vi "TestAdministrator.vi"() -> ()   [LabVIEW 2017]
doc: "Test executive administrator."
uses:
  Shared/Support_InvocationInfo.ctl
panel:
  out "error out":errorcluster
  out "Allocated Memory":T1(graph)
  out "PASS":bool
  in  "Unload after sequence done?":bool
  out "Sequence start time":string
  in  "Only save fails?":bool
  out "# of steps PASSED":i32
  out "# of steps executed":i32
  out "Result file":path
  out "Loop index":i32
  out "Running":bool
  in  "exit":bool
  in  "stop":bool
  out "Last step result":string
  in  "Run":bool
  in  "Nr of loops":i32=1
  in  "Loop infinitive?":bool
  in  "Save to result file?":bool=TRUE
  in  "Result folder":path=path "C:/Users/materi/Documents/G#"
  in  "Load":bool
  in  "Test case folder":path=path "C:/Projects/GsharpGIT2017/Verification/TestCases"
  in  "Sequence file":path=path "C:/Projects/GsharpGIT2017/Verification/TestCases/KernelTestSequence.seq"
  out "Steps":i32(listbox)
  # "Test Administrator"
  # "Execution"
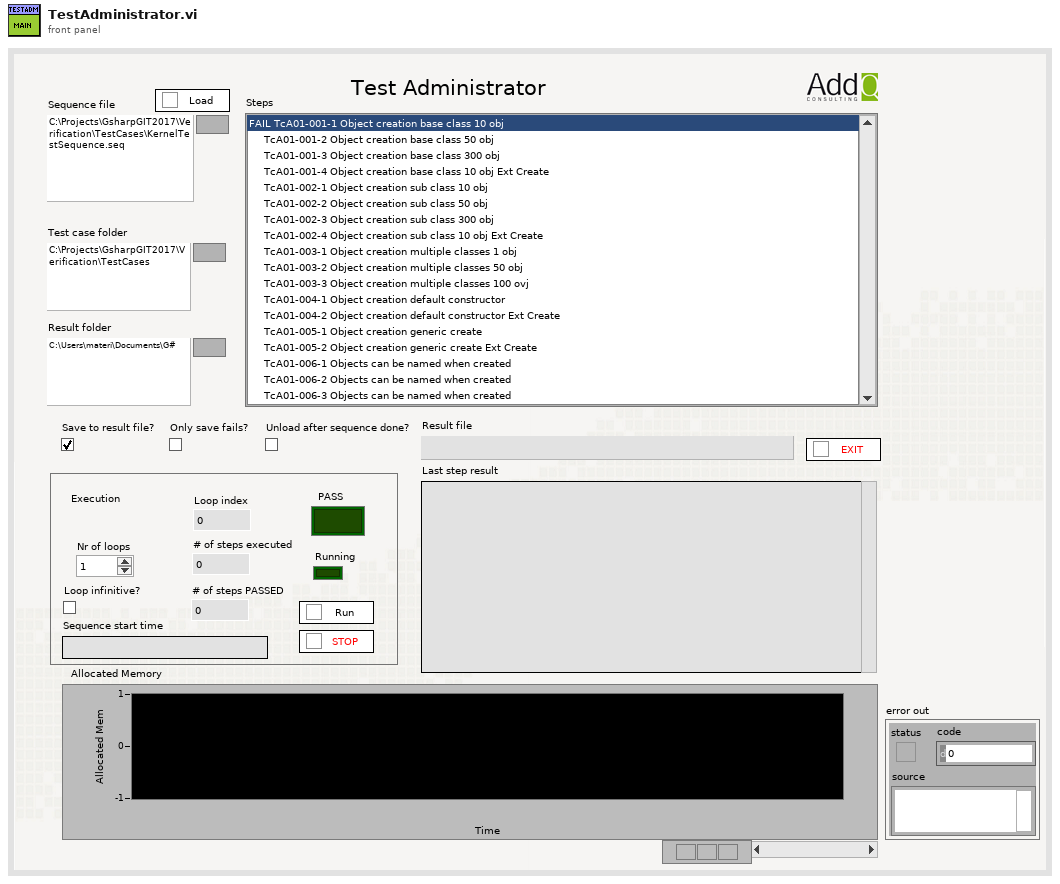
[diagram p1: front panel]
types:
  T1 = cluster{"seconds since 1Jan1904":timestamp, "totAllocSize":i64}[]
  T2 = cluster{"Step names":string[], "Step VIs":string[], "Input Buffer":string[], "Step VI paths":path[], "Loop infinite":bool, "Sequence start time":string, "Save to result file?":bool, "Result file":refnum<file>, "File index":i32, "Nr of PASS":i32, "Nr of steps":i32}
  T3 = enum16{"open", "open or create", "create or replace", "create", "open (read only)"}
  T4 = typedef "Support_InvocationInfo.ctl" = cluster{"UUT #":i32, "loop #":i32, "UUT Info":string, "Test Name":string, "Sequence Path":path}
  T5 = cluster{"PASS/FAIL Flag":bool, "Numeric Measurement":dbl, "String Measurement":string, "Report Text":string}
  T6 = cluster{"totalFreeSize":i64, "maxFreeSize":i64, "nFreeblocks":i64, "totAllocSize":i64, "maxAllocSize":i64, "nPointers":i64, "nUnlockedHdls":i64, "nLockedHdls":i64, "reserved1":i32, "reserved2":i32, "reserved3":i32, "reserved4":i32}
  T7 = cluster{"seconds since 1Jan1904":timestamp, "totAllocSize":i64}
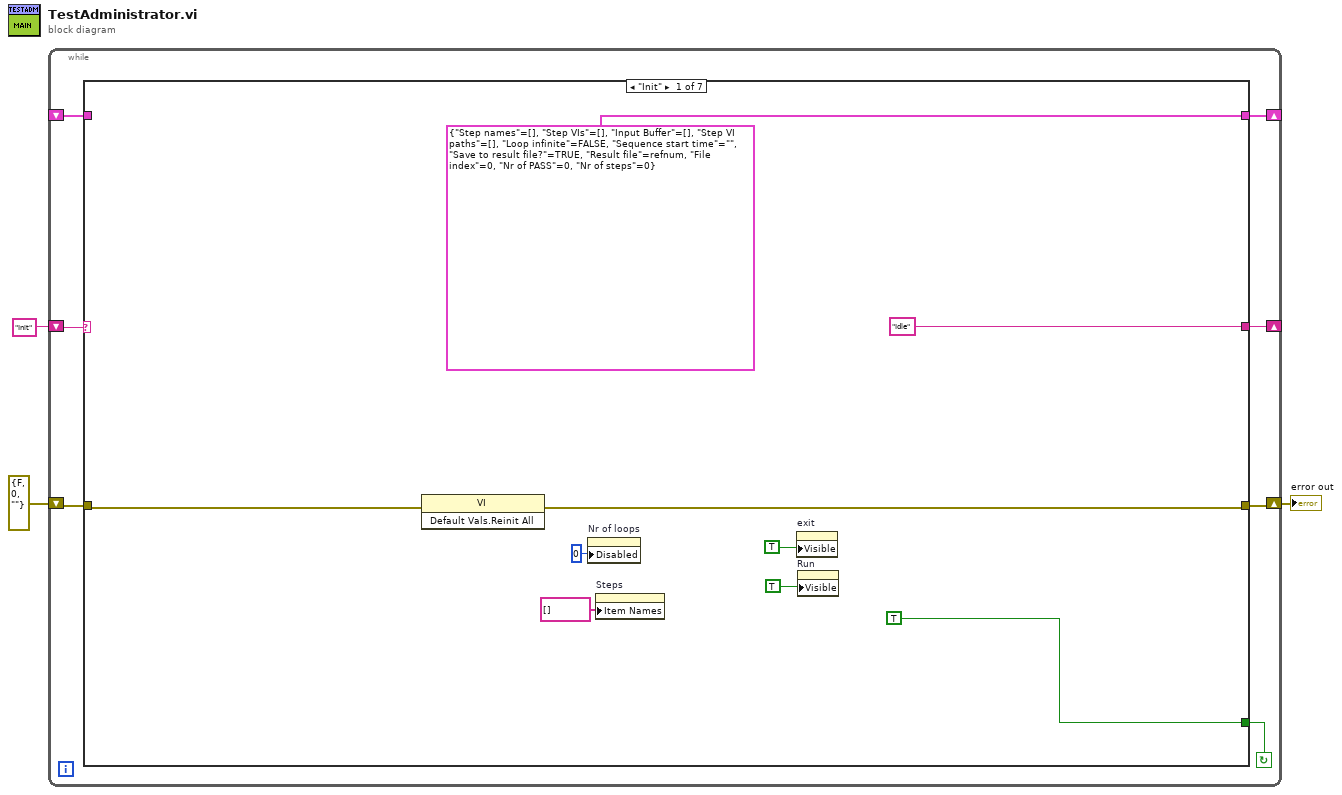
[diagram p0: block diagram]
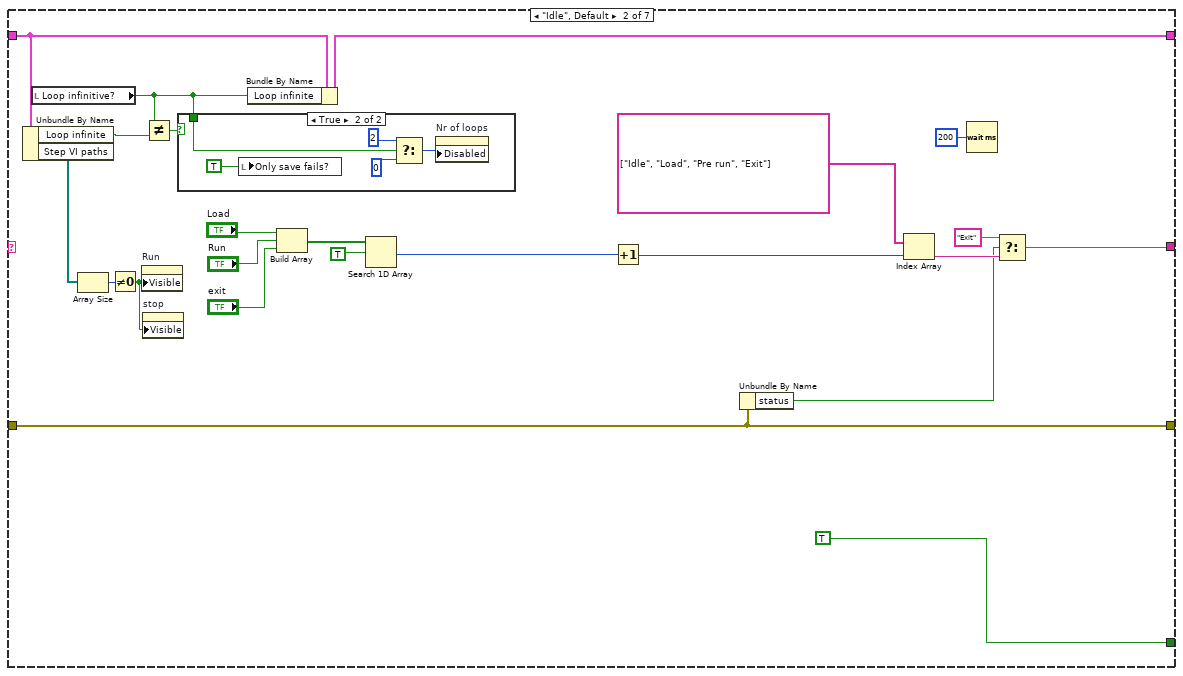
[diagram p2: hidden frame]
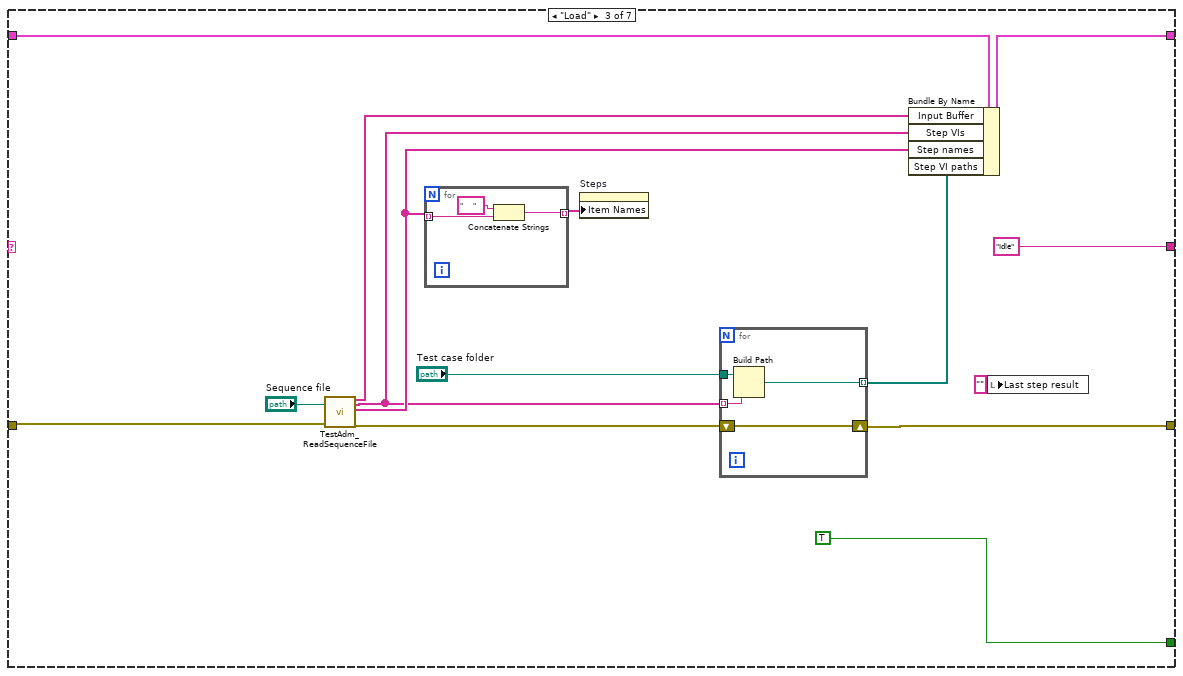
[diagram p4: hidden frame]
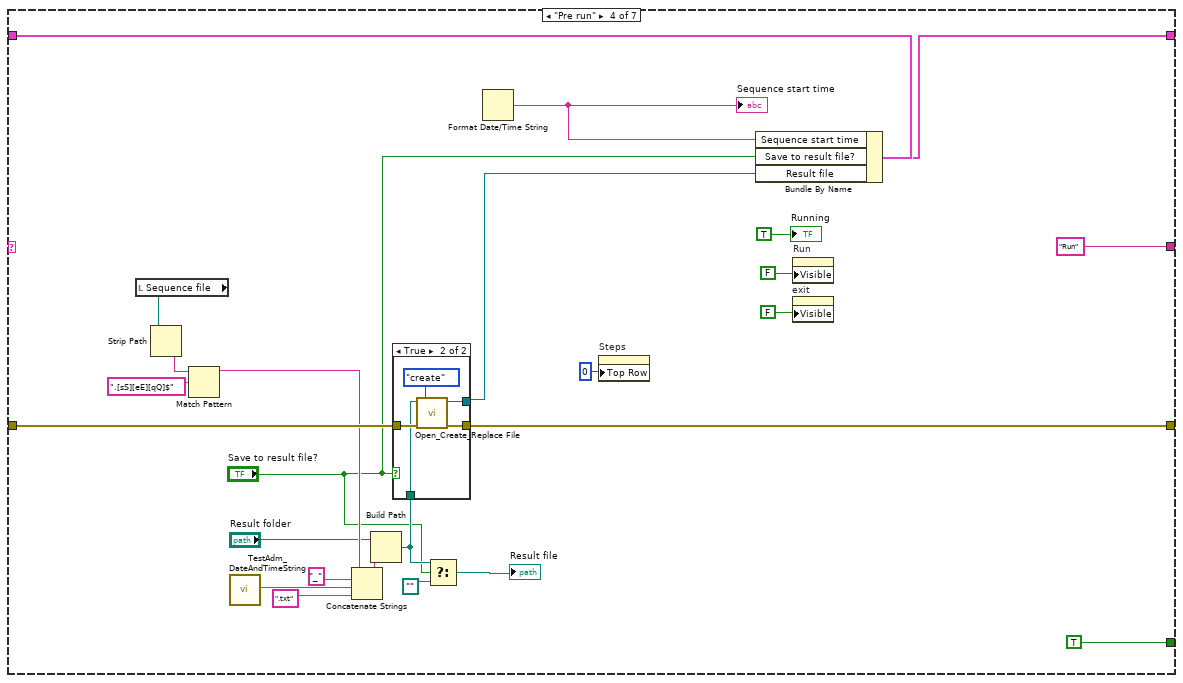
[diagram p5: hidden frame]
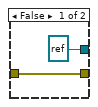
[diagram p6: hidden frame]
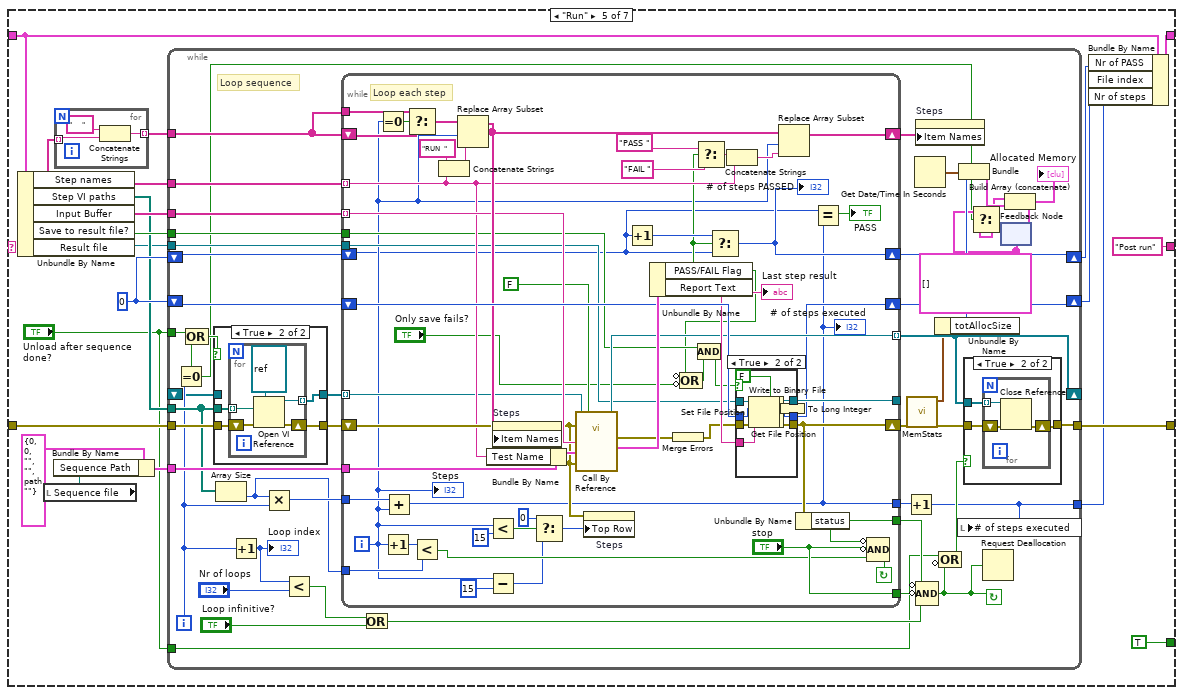
[diagram p7: hidden frame]
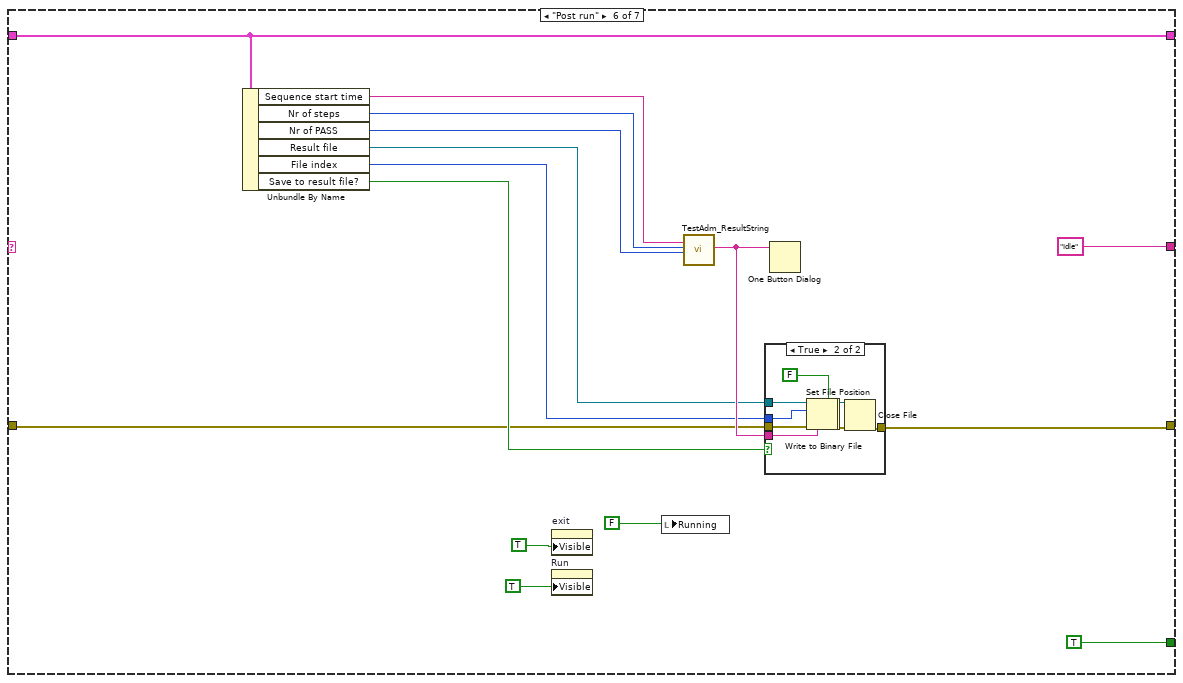
[diagram p11: hidden frame]
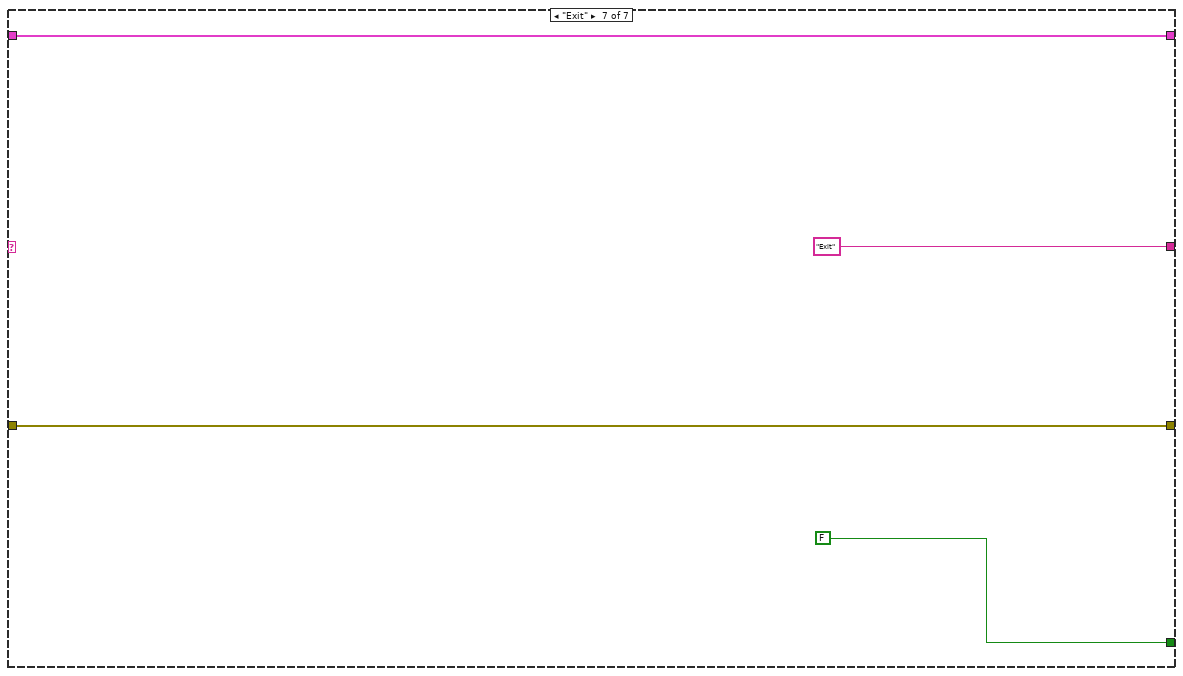
[diagram p13: hidden frame]
diagram:
  n1 = while {
    shift-left: errorcluster {"status"=FALSE, "code"=0, "source"=""} ("error out") -> [w8]
    shift-right: [w7] -> w1
    shift-left: _ -> [w6]
    shift-right: [w9] -> _
    shift-left: "Init" -> [w10]
    shift-right: [w5] -> _
    stop <- w4 continue-if-true
    n2 = case shown="\"Init\"" w10 {
      tunnel: [T2 {"Step names"=[], "Step VIs"=[], "Input Buffer"=[], "Step VI paths"=[], "Loop infinite"=FALSE, "Sequence start time"="", "Save to result file?"=TRUE, "Result file"=refnum, "File index"=0, "Nr of PASS"=0, "Nr of steps"=0} w26 w61 w77 w110 w267 w286] -> w9
      tunnel: w8 -> [w17 w31 w49 w92 w113 w262 w285]
      tunnel: [w16 w31 w56 w79 w112 w269 w285] -> w7
      tunnel: w6 -> [_ w27 w57 w78 w111 w267 w286]
      tunnel: ["Idle" w34 "Idle" "Run" ("t") "Post run" ("t") "Idle" ("t") "Exit" ("t")] -> w5
      tunnel: [TRUE TRUE TRUE TRUE TRUE TRUE FALSE] -> w4
      frame "Init" {
        n3 = invoke class="VI" method="Default Vals.Reinit All"(error in=w17) -> (error out=w16:errorcluster)  [unwired: 2 in, 2 out]
        n4 = property on="Nr of loops" class="DigNum (strict)"("Disabled"=u8 0) -> ()  [unwired: 2 in, 2 out]
        n5 = property on="Steps" class="LstBox (strict)"("Item Names"=string[] []) -> ()  [unwired: 2 in, 2 out]
        n6 = property on="exit" class="Bool"("Visible"=TRUE) -> ()  [unwired: 2 in, 2 out]
        n7 = property on="Run" class="Bool"("Visible"=TRUE) -> ()  [unwired: 2 in, 2 out]
      }
      frame "Idle", Default {
        n8 = Unbundle By Name(w27) -> ("Loop infinite"=w25:bool, "Step VI paths"=w23:path[])
        n9 = local read "Loop infinitive?"() -> (w20:bool)
        n10 = Array Size(array=w23) -> (size(s)=w22:i32)
        n11 = Not Equal To 0?(x=w22) -> (x != 0?=w21:bool)
        n12 = property on="Run" class="Bool"("Visible"=w21) -> ()  [unwired: 2 in, 2 out]
        n13 = property on="stop" class="Bool"("Visible"=w21) -> ()  [unwired: 2 in, 2 out]
        n14 = Not Equal?(x=w20, y=w25) -> (x != y?=w24:bool)
        n15 = case shown="True" w24 {
          tunnel: w20 -> [_ w46]
          frame False {
          }
          frame True {
            n16 = local write "Only save fails?"(TRUE ("Save to result file?")) -> ()
            n17 = Select(t=u8 2 ("Disabled"), s=w46, f=u8 0 ("Disabled")) -> (s? t:f=w43:u8)
            n18 = property on="Nr of loops" class="DigNum (strict)"("Disabled"=w43) -> ()  [unwired: 2 in, 2 out]
          }
        }
        n19 = Bundle By Name(cluster=w27, "Loop infinite"=w20) -> (w26:T2)
        n20 = Build Array("Load", "Run", "exit") -> (w35:bool[])
        n21 = Search 1D Array(1D array=w35, element=TRUE) -> (index of element=w40:i32)  [unwired: 1 in]
        n22 = Increment(x=w40) -> (x+1=w41:i32)
        n23 = Unbundle By Name(w31) -> ("status"=w30:bool)
        n24 = Index Array(array=string[] ["Idle", "Load", "Pre run", "Exit"] ("Array Constant"), index=w41) -> (element=w33:string)
        n25 = Wait (ms)(milliseconds to wait=u32 200) -> ()  [unwired: 1 out]
        n26 = Select(t="Exit", s=w30, f=w33) -> (s? t:f=w34:string)
      }
      frame "Load" {
        n27 = call "TestAdm_ReadSequenceFile.vi"("Path"="Sequence file", "error in (no error)"=w49) -> ("Input Buffer"=w60:string[], "Step paths"=w50:string[], "Step names"=w52:string[], "error out"=w55:errorcluster)  [unwired: 14 in]
        n28 = for {
          tunnel: [w63] -> w53 mode=indexing
          tunnel: w52 -> [w65] mode=indexing
          n29 = Concatenate Strings("     " ("Substring"), w65) -> (w63:string)
        }
        n30 = property on="Steps" class="LstBox (strict)"("Item Names"=w53) -> ()  [unwired: 2 in, 2 out]
        n31 = for {
          shift-right: [w67] -> w56
          shift-left: w55 -> [w67]
          tunnel: "Test case folder" -> [w69]
          tunnel: w50 -> [w68] mode=indexing
          tunnel: [w66] -> w48 mode=indexing
          n32 = Build Path(base path=w69, name or relative path=w68) -> (appended path=w66:path)
        }
        n33 = Bundle By Name(cluster=w57, "Input Buffer"=w60, "Step VIs"=w50, "Step names"=w52, "Step VI paths"=w48) -> (w61:T2)
        n34 = local write "Last step result"("" ("Last Step result")) -> ()
      }
      frame "Pre run" {
        n35 = local read "Sequence file"() -> (w87:path)
        n36 = Strip Path(path=w87) -> (name=w86:string)  [unwired: 1 out]
        n37 = Match Pattern(string=w86, regular expression=".[sS][eE][qQ]$") -> (before substring=w85:string)  [unwired: 1 in, 3 out]
        n38 = call "TestAdm_DateAndTimeString.vi"() -> ("String out"=w91:string)  [unwired: 19 in]
        n39 = Concatenate Strings(w85, "_", w91, ".txt" ("Substring")) -> (w90:string)
        n40 = Build Path(base path="Result folder", name or relative path=w90) -> (appended path=w89:path)
        n41 = case shown="True" "Save to result file?" {
          tunnel: w92 -> [w96 w101]
          tunnel: [refnum<file> refnum ("refnum") w100] -> w74
          tunnel: [w96 w99] -> w79
          tunnel: w89 -> [_ w97]
          frame False {
          }
          frame True {
            n42 = call <vilib>:"Open_Create_Replace File.vi"("error in (no error)"=w101, "function (open:0)"=T3."create", "file path"=w97) -> ("error out"=w99:errorcluster, "refnum"=w100:refnum<file>)  [unwired: 5 in, 2 out]
          }
        }
        n43 = Select(t=w89, s="Save to result file?", f=path "") -> (s? t:f=→"Result file":path)
        n44 = Format Date/Time String() -> (date/time string=w76:string)  [unwired: 3 in]
        "Sequence start time" <- w76
        n45 = property on="Steps" class="LstBox (strict)"("Top Row"=0) -> ()  [unwired: 2 in, 2 out]
        n46 = Bundle By Name(cluster=w78, "Sequence start time"=w76, "Save to result file?"="Save to result file?", "Result file"=w74) -> (w77:T2)
        n47 = property on="Run" class="Bool"("Visible"=FALSE) -> ()  [unwired: 2 in, 2 out]
        n48 = property on="exit" class="Bool"("Visible"=FALSE) -> ()  [unwired: 2 in, 2 out]
        "Running" <- TRUE ("Running")
      }
      frame "Run" {
        w107 = 0 ("offset")
        n49 = Unbundle By Name(w111) -> ("Step names"=w117:string[], "Step VI paths"=w106:path[], "Input Buffer"=w109:string[], "Save to result file?"=w114:bool, "Result file"=w105:refnum<file>)
        n50 = local read "Sequence file"() -> (w115:path)
        n51 = Bundle By Name(cluster=T4 {"UUT #"=0, "loop #"=0, "UUT Info"="", "Test Name"="", "Sequence Path"=path ""} ("Invocation info"), "Sequence Path"=w115) -> (w118:T4)
        n52 = for {
          tunnel: w117 -> [w258] mode=indexing
          tunnel: [w256] -> w116 mode=indexing
          n53 = Concatenate Strings("     ", w258) -> (w256:string)
        }
        n54 = while {
          tunnel: [w134] -> w102
          shift-left: _ -> [w137]
          shift-right: [w136] -> _
          tunnel: "Unload after sequence done?" -> [w138]
          tunnel: "Unload after sequence done?" -> [w139]
          tunnel: w105 -> [w154]
          tunnel: w106 -> [w153]
          shift-left: w107 -> [w158]
          shift-right: [w160] -> w108
          shift-left: w107 -> [w159]
          shift-right: [w161] -> w103
          tunnel: [w142] -> w112
          tunnel: w113 -> [w156]
          tunnel: w114 -> [w162]
          tunnel: w116 -> [w163]
          tunnel: w117 -> [w164]
          tunnel: w109 -> [w166]
          tunnel: w118 -> [w167]
          i -> [w141]
          stop <- w130 continue-if-true
          w125 = T1 []
          # "Loop sequence"
          n55 = Equal To 0?(x=w141) -> (x = 0?=w122:bool)
          n56 = Compound Arithmetic op=OR(w139, w122) -> (w140:bool)
          n57 = case shown="True" w140 {
            tunnel: [w246 w250] -> w157
            tunnel: w156 -> [w246 w249]
            tunnel: [w245 w248] -> w155
            tunnel: w153 -> [_ w247]
            tunnel: w137 -> [w245 _]
            frame False {
            }
            frame True {
              n58 = for {
                shift-right: [w254] -> w250
                shift-left: w249 -> [w255]
                tunnel: [w252] -> w248 mode=indexing
                tunnel: w247 -> [w251] mode=indexing
                n59 = Open VI Reference(type specifier VI Refnum (for type only)=refnum<vi> refnum ("VI Refnum"), vi path=w251, error in (no error)=w255) -> (vi reference=w252:refnum<vi>, error out=w254:errorcluster)  [unwired: 3 in]
              }
            }
          }
          n60 = Array Size(array=w153) -> (size(s)=w148:i32)
          n61 = Increment(x=w141) -> (x+1=w147:i32)
          "Loop index" <- w147
          n62 = Multiply(x=w148, y=w141) -> (x*y=w152:i32)
          n63 = Less?(x=w147, y="Nr of loops") -> (x < y?=w145:bool)
          n64 = while {
            tunnel: w148 -> [w189]
            tunnel: ["stop"] -> w149
            tunnel: [w221] -> w150
            tunnel: [w171] -> w151
            tunnel: w152 -> [w191]
            tunnel: w154 -> [w192]
            tunnel: [w193] -> w136 mode=indexing
            tunnel: w155 -> [w194] mode=indexing
            tunnel: w163 -> [w199]
            shift-left: w159 -> [w169]
            shift-right: [w173] -> w161
            shift-left: w163 -> [w200]
            shift-right: [w214] -> w165
            tunnel: w164 -> [w195] mode=indexing
            tunnel: [w215] -> _
            shift-left: w158 -> [w217]
            shift-right: [w172] -> w160
            tunnel: w162 -> [w178]
            tunnel: w166 -> [w196] mode=indexing
            tunnel: w167 -> [w209]
            shift-left: w157 -> [w204]
            shift-right: [w218] -> w133
            i -> [w170]
            stop <- w220 continue-if-true
            # "Loop each step"
            n65 = Equal To 0?(x=w170) -> (x = 0?=w197:bool)
            n66 = Increment(x=w170) -> (x+1=w175:i32)
            n67 = Add(x=w191, y=w170) -> (x+y=w171:i32)
            "# of steps executed" <- w171
            n68 = Select(t=w199, s=w197, f=w200) -> (s? t:f=w198:string[])
            n69 = Less?(x=w175, y=w189) -> (x < y?=w188:bool)
            n70 = Concatenate Strings("RUN  ", w195) -> (w205:string)
            n71 = Replace Array Subset(array=w198, new element=w205, index=w170) -> (w207:string[])
            n72 = Bundle By Name(cluster=w209, "Test Name"=w195) -> (w208:T4)
            n73 = Less?(x=w170, y=15) -> (x < y?=w186:bool)
            n74 = Subtract(x=w170, y=15) -> (x-y=w182:i32)
            n75 = property on="Steps" class="LstBox (strict)"(error in=w204, "Item Names"=w207) -> (error out=w181:errorcluster)  [unwired: 1 in, 1 out]
            n76 = Select(t=0 ("y"), s=w186, f=w182) -> (s? t:f=w187:i32)
            n77 = call-by-ref "?"(reference=w194, error in=w181, "Input buffer"=w196, "Invocation info"=w208, "error in (no error)"=w181, "Add log to result?"=FALSE) -> (reference out=w193:refnum<vi>, error out=w202:errorcluster, "Test Data"=w219:T5)  [unwired: 14 in, 1 out]
            n78 = property on="Steps" class="LstBox (strict)"(error in=w181, "Top Row"=w187) -> ()  [unwired: 1 in, 2 out]
            n79 = Increment(x=w169) -> (x+1=w203:i32)
            n80 = Unbundle By Name(w219) -> ("PASS/FAIL Flag"=w176:bool, "Report Text"=w216:string)
            "Last step result" <- w216
            n81 = Merge Errors(w202) -> (w201:errorcluster)
            n82 = Compound Arithmetic op=OR(invert w176, invert "Only save fails?") -> (w177:bool)
            n83 = Select(t="PASS ", s=w176, f="FAIL ") -> (s? t:f=w211:string)
            n84 = Compound Arithmetic op=AND(w178, w177) -> (w179:bool)
            n85 = Select(t=w203, s=w176, f=w169) -> (s? t:f=w173:i32)
            "# of steps PASSED" <- w173
            n86 = Concatenate Strings(w211, w195) -> (w210:string)
            n87 = case shown="True" w179 {
              tunnel: w201 -> [w222 w237]
              tunnel: [w222 w236] -> w218
              tunnel: w192 -> [w223 w235]
              tunnel: w217 -> [w224 w234]
              tunnel: [w224 w233] -> w172
              tunnel: w216 -> [_ w232]
              tunnel: [w223 w231] -> w215
              frame False {
              }
              frame True {
                n88 = Set File Position(offset (in bytes) (0)=w234, refnum=w235, error in=w237) -> (refnum out=w230:refnum<file>, error out=w229:errorcluster)  [unwired: 1 in]
                n89 = Write to Binary File(file (use dialog)=w230, data=w232, error in=w229, 5:FALSE ("prepend array or string size? (T)")) -> (refnum out=w228:refnum<file>, error out=w227:errorcluster)  [unwired: 2 in, 1 out]
                n90 = Get File Position(4:w227, 7:w228) -> (0:w236:errorcluster, 2:w226:i64, 3:w231:refnum<file>)
                n91 = To Long Integer(number=w226) -> (32bit integer=w233:i32)
              }
            }
            n92 = Replace Array Subset(array=w207, new element=w210, index=w170) -> (w214:string[])
            n93 = Unbundle By Name(w218) -> ("status"=w221:bool)
            n94 = Equal?(x=w169, y=w171) -> (x = y?=→"PASS":bool)
            n95 = Compound Arithmetic op=AND(invert w221, invert "stop", w188) -> (w220:bool)
            "Steps" <- w170
          }
          n96 = Or(x=w145, y="Loop infinitive?") -> (x .or. y?=w143:bool)
          n97 = Increment(x=w151) -> (x+1=w134:i32)
          n98 = call <vilib>:"MemStats.vi"("error in"=w133) -> ("error out"=w132:errorcluster, "AZ memStats"=w131:T6)  [unwired: 4 in, 1 out]
          n99 = Get Date/Time In Seconds() -> (seconds since 1Jan1904=w129:timestamp)
          n100 = property on="Steps" class="LstBox (strict)"("Item Names"=w165) -> ()  [unwired: 2 in, 2 out]
          n101 = Compound Arithmetic op=AND(invert w150, invert w149, w143) -> (w130:bool)
          n102 = Unbundle By Name(w131) -> ("totAllocSize"=w128:i64)
          n103 = Compound Arithmetic op=OR(w138, invert w130) -> (w135:bool)
          n104 = local write "# of steps executed"(w134) -> ()
          n105 = Bundle("seconds since 1Jan1904"=w129, "totAllocSize"=w128) -> (w127:T7)  [unwired: 1 in]
          n106 = case shown="True" w135 {
            tunnel: w132 -> [w238 w241]
            tunnel: w136 -> [_ w240]
            tunnel: [w238 w239] -> w142
            frame False {
            }
            frame True {
              n107 = for {
                shift-right: [w243] -> w239
                shift-left: w241 -> [w244]
                tunnel: w240 -> [w242] mode=indexing
                n108 = Close Reference(reference=w242, error in (no error)=w244) -> (error out=w243:errorcluster)
              }
            }
          }
          n109 = Request Deallocation(w130) -> ()
          n110 = feedback #1(w125) -> (w124:T1)
          n111 = Select(t=w125, s=w122, f=w124) -> (s? t:f=w123:T1)
          n112 = Build Array (concatenate)(w123, w127) -> (w126:T1)
          "Allocated Memory" <- w126
          n113 = feedback-in #1(w126) -> ()
        }
        n114 = Bundle By Name(cluster=w111, "Nr of PASS"=w103, "File index"=w108, "Nr of steps"=w102) -> (w110:T2)
      }
      frame "Post run" {
        n115 = Unbundle By Name(w267) -> ("Sequence start time"=w266:string, "Nr of steps"=w260:i32, "Nr of PASS"=w259:i32, "Result file"=w265:refnum<file>, "File index"=w264:i32, "Save to result file?"=w263:bool)
        n116 = property on="exit" class="Bool"("Visible"=TRUE) -> ()  [unwired: 2 in, 2 out]
        n117 = property on="Run" class="Bool"("Visible"=TRUE) -> ()  [unwired: 2 in, 2 out]
        n118 = local write "Running"(FALSE ("Running")) -> ()
        n119 = call "TestAdm_ResultString.vi"("Sequence start time"=w266, "Nr of steps"=w260, "Nr of PASS"=w259) -> ("Result string"=w271:string)  [unwired: 16 in]
        n120 = case shown="True" w263 {
          tunnel: [w274 w284] -> w269
          tunnel: w262 -> [w274 w283]
          tunnel: w265 -> [_ w282]
          tunnel: w264 -> [_ w279]
          tunnel: w271 -> [_ w278]
          frame False {
          }
          frame True {
            n121 = Set File Position(offset (in bytes) (0)=w279, refnum=w282, error in=w283) -> (refnum out=w277:refnum<file>, error out=w276:errorcluster)  [unwired: 1 in]
            n122 = Write to Binary File(file (use dialog)=w277, data=w278, error in=w276, 5:FALSE ("prepend array or string size? (T)")) -> (refnum out=w281:refnum<file>, error out=w280:errorcluster)  [unwired: 2 in, 1 out]
            n123 = Close File(refnum=w281, error in=w280) -> (error out=w284:errorcluster)  [unwired: 1 out]
          }
        }
        n124 = One Button Dialog(message=w271) -> ()  [unwired: 1 in, 1 out]
      }
      frame "Exit" {
      }
    }
  }
  "error out" <- w1
